vi "Configure Bus Monitor.vi"(8 "error in (no error)":errorcluster) -> (0 "error out":errorcluster, 3 "Bus Monitor":refnum<class "Bus Monitor.lvclass">)   [LabVIEW 2020, in "BCI-1553 RealTime API Examples.lvlib"]
uses:
  BCI-1553 RealTime API Examples.lvlib
  src/RealTime/Bus Monitor/Bus Monitor.lvclass
  src/RealTime/Bus Monitor/TypeDefs/Bus Monitor Configuration.ctl
  src/RealTime/Bus Monitor/TypeDefs/Bus Monitor Timeout.ctl
  src/RealTime/Bus Monitor/TypeDefs/Bus Monitor Timetag Behavior.ctl
  src/RealTime/Bus Monitor/TypeDefs/Bus Monitor Record Requirement.ctl
  src/RealTime/Bus Monitor/TypeDefs/Bus Monitor Timetag Configuration.ctl
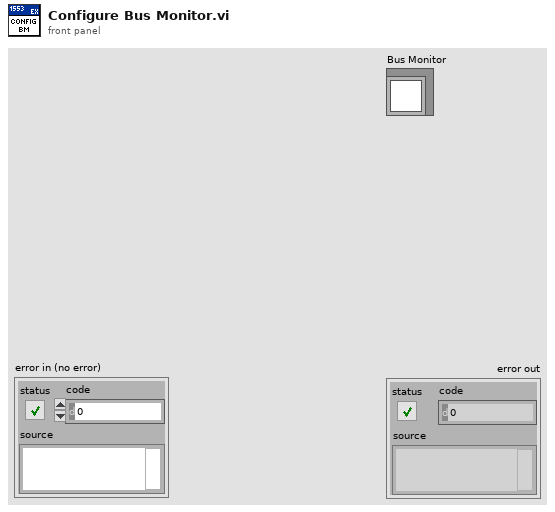
[diagram p1: front panel]
types:
  T1 = typedef "BCI-1553 API.lvlib/Bus Monitor.lvclass/Bus Monitor Timetag Configuration.ctl" = enum16{"Disabled", "2us", "4us", "8us", "16us", "32us", "64us", "100ns"}
  T2 = typedef "BCI-1553 API.lvlib/Bus Monitor.lvclass/Bus Monitor Record Requirement.ctl" = enum16{"Properly Encoded - Complete - Cmd Sync", "Properly Encoded - Complete - Cmd or Data Sync", "Properly Encoded Cmd Sync - At Least 2 Data Bits ", "Any Properly Encoded Sync - At Least 2 Data Bits"}
  T3 = typedef "BCI-1553 API.lvlib/Bus Monitor.lvclass/Bus Monitor Timetag Behavior.ctl" = enum16{"Last Bit of Last Word", "First Bit of Command Word", "Last Bit of Command Word", "Timetag Disabled"}
  T4 = typedef "BCI-1553 API.lvlib/Bus Monitor.lvclass/Bus Monitor Timeout.ctl" = enum16{"18us", "23us", "82us", "140us"}
  T5 = typedef "BCI-1553 API.lvlib/Bus Monitor.lvclass/Bus Monitor Configuration.ctl" = cluster{"Timeout":T4, "Gap Check":bool, "Timetag Behavior":T3, "Record Requirement":T2, "Cont Record After Inv Word":bool, "Ext Msg Flag Enable":bool, "48-bit Time Tag":bool, "Simple Mode":bool, "Bus Monitor Timetag Config":T1}
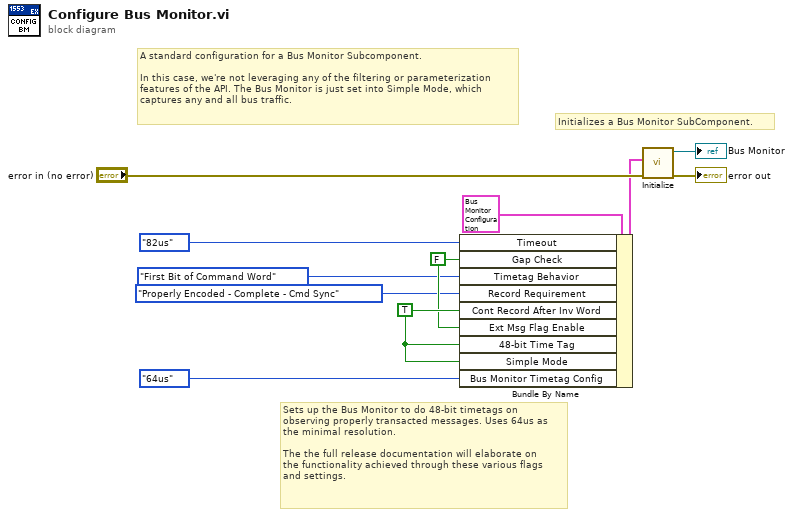
[diagram p0: block diagram]
diagram:
  w5 = TRUE ("Cont Record After Inv Word")
  w4 = FALSE ("Gap Check")
  # "Initializes a Bus Monitor SubComponent."
  # "Sets up the Bus Monitor to do 48-bit timetags on \nobserving properly transacted messages. Uses 64us as\nthe minimal resolution.\n\nThe the full release documentation will elaborate on\nthe functionality achieved through these various flags\nand settings."
  # "A standard configuration for a Bus Monitor Subcomponent.\n\nIn this case, we're not leveraging any of the filtering or parameterization\nfeatures of the API. The Bus Monitor is just set into Simple Mode, which\ncaptures any and all bus traffic."
  n1 = Bundle By Name(cluster=T5 {"Timeout"=enum."18us", "Gap Check"=FALSE, "Timetag Behavior"=enum."Last Bit of Last Word", "Record Requirement"=enum."Properly Encoded - Complete - Cmd Sync", "Cont Record After Inv Word"=FALSE, "Ext Msg Flag Enable"=FALSE, "48-bit Time Tag"=FALSE, "Simple Mode"=FALSE, "Bus Monitor Timetag Config"=enum."Disabled"} ("Bus Monitor Configuration"), "Timeout"=Bus_Monitor_Timeout."82us", "Gap Check"=w4, "Timetag Behavior"=Bus_Monitor_Timetag_Behavior."First Bit of Command Word", "Record Requirement"=Bus_Monitor_Record_Requirement."Properly Encoded - Complete - Cmd Sync", "Cont Record After Inv Word"=w5, "Ext Msg Flag Enable"=w4, "48-bit Time Tag"=w5, "Simple Mode"=w5, "Bus Monitor Timetag Config"=Bus_Monitor_Timetag_Configuration."64us") -> (w7:T5)
  n2 = call "Initialize.vi"("error in (no error)"="error in (no error)", "Bus Monitor Configuration"=w7) -> ("error out"=→"error out":errorcluster, "Bus Monitor out"=→"Bus Monitor":refnum<class "Bus Monitor.lvclass">)  [unwired: 8 in]
